vi "Self-Calibrate.vi"(6 "Remote Timeout (300,000 ms)":u32=300000, 8 "error in (no error)":errorcluster, 11 "Resource in":refnum<k20>) -> (0 "error out":errorcluster, 2 "Detailed Result":string, 3 "Resource out":refnum<k20>)   [LabVIEW 2012, in "nisyscfg.lvlib"]
doc: "Performs a self-calibration on a device. Self-calibration adjusts the calibration constants with respect to an onboard reference stored on the device. The new calibration constants are defined with respect to the calibration constants created during an external calibration to ensure that the measurements are traceable to these external standards. The new calibration constants do not affect the constants created during an external calibration because they are stored in a different area of the device memory. You can perform a self-calibration at any time to adjust the device for use in environments other than those in which the device was externally calibrated."
uses:
  <vilib>/nisyscfg/nisyscfg.lvlib
  <vilib>/Utility/error.llb/Error Cluster From Error Code.vi
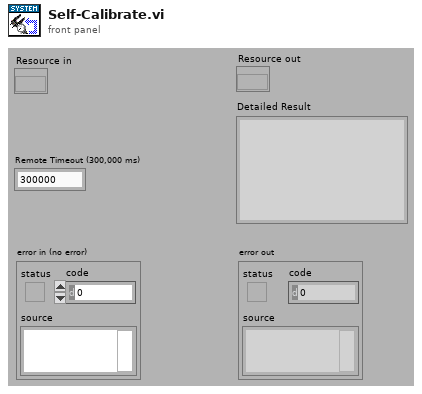
[diagram p1: front panel]
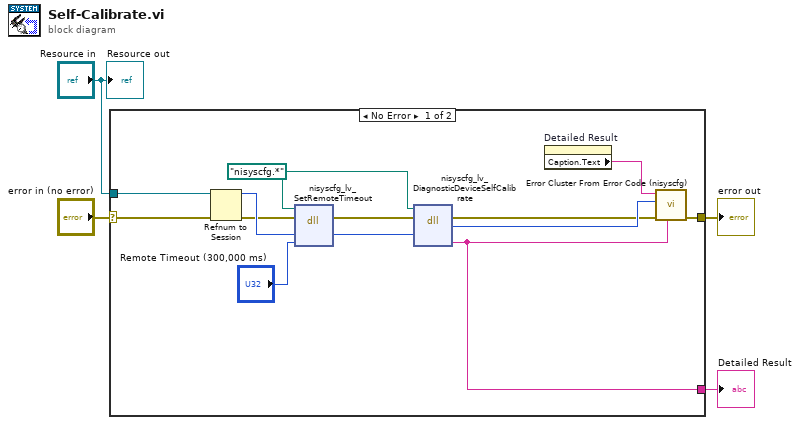
[diagram p0: block diagram]
diagram:
  n1 = case shown="No Error" "error in (no error)" {
    selector: "error in (no error)" -> [w9 w18]
    tunnel: [w15 w18] -> w4
    tunnel: "Resource in" -> [w8 _]
    tunnel: [w5 _] -> w1
    frame No Error {
      w7 = path "nisyscfg.*" ("path in")
      n2 = Refnum to Session(4:w9, 7:w8) -> (0:w12:errorcluster, 3:w13:u64)
      n3 = dll-call lib="nisyscfg.*" fn="nisyscfg_lv_SetRemoteTimeout" label="SetRemoteTimeout"(path in=w7, error in=w12, "item"=w13, "connectTimeout"="Remote Timeout (300,000 ms)") -> (error out=w11:errorcluster, "item"=w10:u64)  [unwired: 1 in, 3 out]
      n4 = dll-call lib="nisyscfg.*" fn="nisyscfg_lv_DiagnosticDeviceSelfCalibrate" label="DiagnosticDeviceSelfCalibrate"(path in=w7, error in=w11, "item"=w10) -> (error out=w16:errorcluster, "status"=w17:i32, "detailed result"=w5:string)  [unwired: 1 in, 3 out]
      n5 = property on="Detailed Result" class="Str"() -> ("Caption.Text"=w6:string)  [unwired: 2 in, 2 out]
      n6 = call <vilib>:"Error Cluster From Error Code (nisyscfg).vi"("Details String"=w5, "error in (no error)"=w16, "Error Code (0)"=w17, "Details Caption"=w6) -> ("error out"=w15:errorcluster)  [unwired: 7 in]
    }
    frame Error {
    }
  }
  "error out" <- w4
  "Detailed Result" <- w1
  "Resource out" <- "Resource in"
